vi "Chameleon Prompt Echo Off.vi"(0 "VISA Ref":refnum<visa-resource-name>, 11 "Error In":errorcluster) -> (4 "VISA Ref Out":refnum<visa-resource-name>, 15 "Error Out":errorcluster)   [LabVIEW 2020]
panel:
  out "Response 02":string
  out "Response 01":string
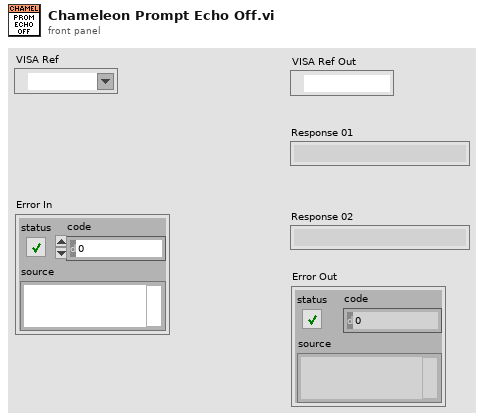
[diagram p1: front panel]
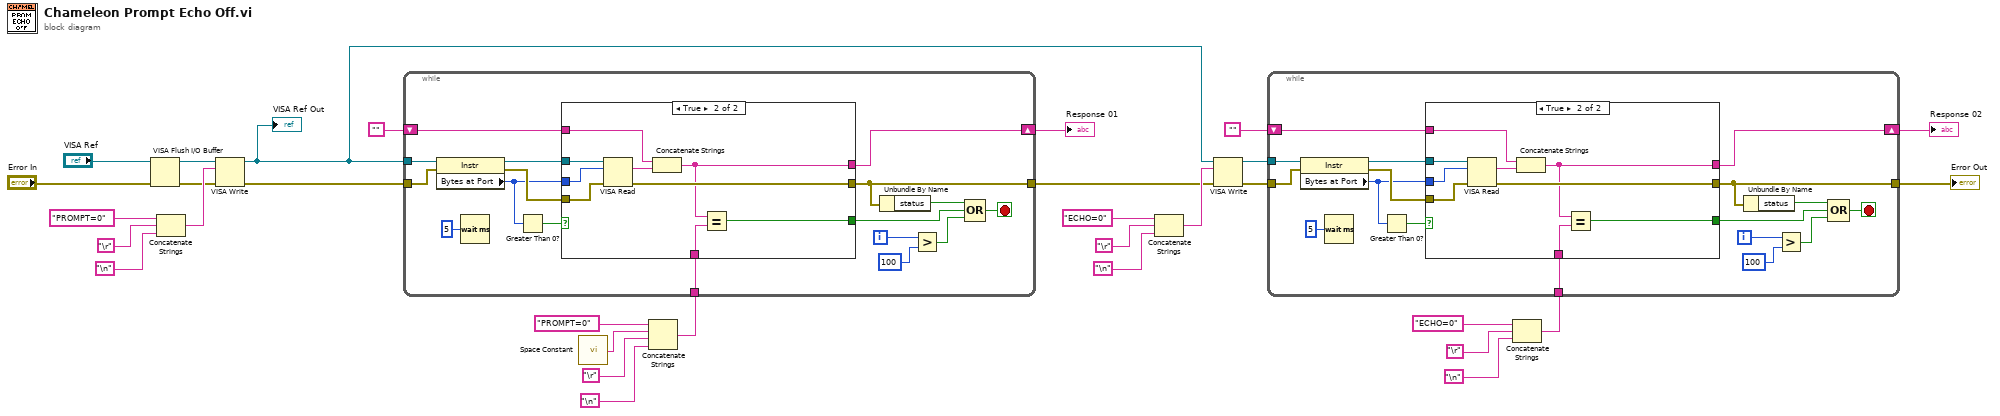
[diagram p0: block diagram]
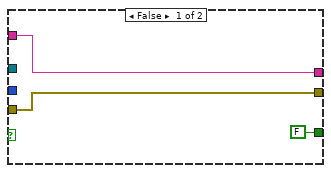
[diagram p2: hidden frame]
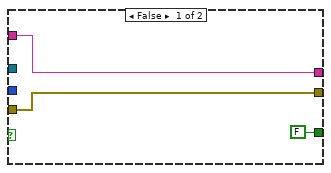
[diagram p3: hidden frame]
diagram:
  n1 = VISA Flush I/O Buffer(VISA resource name="VISA Ref", error in (no error)="Error In") -> (VISA resource name out=w24:refnum<visa-resource-name>, error out=w22:errorcluster)  [unwired: 1 in]
  n2 = Concatenate Strings("PROMPT=0" ("Command"), "\r", "\n") -> (w27:string)
  n3 = VISA Write(VISA resource name=w24, write buffer=w27, error in (no error)=w22) -> (VISA resource name out=w4:refnum<visa-resource-name>, error out=w26:errorcluster)  [unwired: 1 out]
  "VISA Ref Out" <- w4
  n4 = call <vilib>:"Space Constant.vi"() -> ("String"=w18:string)
  n5 = Concatenate Strings("PROMPT=0" ("Command"), w18, "\r", "\n") -> (w17:string)
  n6 = while {
    tunnel: w4 -> [w48]
    tunnel: w26 -> [w47]
    shift-right: [w37] -> w2
    shift-left: "" -> [w38]
    tunnel: [w34] -> w5
    tunnel: w17 -> [w32]
    i -> [w46]
    stop <- w44 stop-if-true
    n7 = property class="Instr"(reference=w48, error in=w47) -> (reference out=w40:refnum<visa-resource-name>, error out=w41:errorcluster, "Bytes at Port"=w39:u32)
    n8 = Wait (ms)(milliseconds to wait=u32 5) -> ()  [unwired: 1 out]
    n9 = Greater Than 0?(x=w39) -> (x > 0?=w42:bool)
    n10 = case shown="True" w42 {
      tunnel: w41 -> [w50 w59]
      tunnel: w40 -> [_ w60]
      tunnel: w39 -> [_ w58]
      tunnel: w38 -> [w51 w57]
      tunnel: [w51 w53] -> w37
      tunnel: [w50 w55] -> w34
      tunnel: [FALSE w54] -> w35
      tunnel: w32 -> [_ w52]
      frame False {
      }
      frame True {
        n11 = VISA Read(VISA resource name=w60, byte count=w58, error in (no error)=w59) -> (read buffer=w56:string, error out=w55:errorcluster)  [unwired: 2 out]
        n12 = Concatenate Strings(w57, w56) -> (w53:string)
        n13 = Equal?(x=w53, y=w52) -> (x = y?=w54:bool)
      }
    }
    n14 = Unbundle By Name(w34) -> ("status"=w36:bool)
    n15 = Greater?(x=w46, y=100) -> (0:w33:bool)
    n16 = Compound Arithmetic op=OR(w36, w35, w33) -> (w44:bool)
  }
  "Response 01" <- w2
  n17 = Concatenate Strings("ECHO=0" ("Command"), "\r", "\n") -> (w10:string)
  n18 = VISA Write(VISA resource name=w4, write buffer=w10, error in (no error)=w5) -> (VISA resource name out=w11:refnum<visa-resource-name>, error out=w12:errorcluster)  [unwired: 1 out]
  n19 = Concatenate Strings("ECHO=0" ("Command"), "\r", "\n") -> (w16:string)
  n20 = while {
    tunnel: w11 -> [w77]
    tunnel: w12 -> [w76]
    shift-right: [w66] -> w1
    shift-left: "" -> [w67]
    tunnel: [w63] -> w3
    tunnel: w16 -> [w61]
    i -> [w75]
    stop <- w73 stop-if-true
    n21 = property class="Instr"(reference=w77, error in=w76) -> (reference out=w69:refnum<visa-resource-name>, error out=w70:errorcluster, "Bytes at Port"=w68:u32)
    n22 = Wait (ms)(milliseconds to wait=u32 5) -> ()  [unwired: 1 out]
    n23 = Greater Than 0?(x=w68) -> (x > 0?=w71:bool)
    n24 = case shown="True" w71 {
      tunnel: w70 -> [w79 w88]
      tunnel: w69 -> [_ w89]
      tunnel: w68 -> [_ w87]
      tunnel: w67 -> [w80 w86]
      tunnel: [w80 w82] -> w66
      tunnel: [w79 w84] -> w63
      tunnel: [FALSE w83] -> w64
      tunnel: w61 -> [_ w81]
      frame False {
      }
      frame True {
        n25 = VISA Read(VISA resource name=w89, byte count=w87, error in (no error)=w88) -> (read buffer=w85:string, error out=w84:errorcluster)  [unwired: 2 out]
        n26 = Concatenate Strings(w86, w85) -> (w82:string)
        n27 = Equal?(x=w82, y=w81) -> (x = y?=w83:bool)
      }
    }
    n28 = Unbundle By Name(w63) -> ("status"=w65:bool)
    n29 = Greater?(x=w75, y=100) -> (0:w62:bool)
    n30 = Compound Arithmetic op=OR(w65, w64, w62) -> (w73:bool)
  }
  "Error Out" <- w3
  "Response 02" <- w1
